vi "Read Instant Analog.vi"(10 "Channel":T1, 11 "ADALM2000 Handler":u64 caption="Instrument Handle Out") -> (2 "Read instant analog value":dbl(slide) max=255.0 scale=-25.0..25.0, 3 "ADALM2000 Handler 2":u64 caption="Instrument Handle Out")   [LabVIEW 2022 SP3]
uses:
  Controls/AnalogChannel.ctl
  libm2k_lv.dll
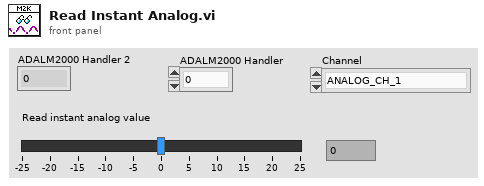
[diagram p1: front panel]
types:
  T1 = typedef "AnalogChannel.ctl" = enum16{"ANALOG_CH_1", "ANALOG_CH_2"}
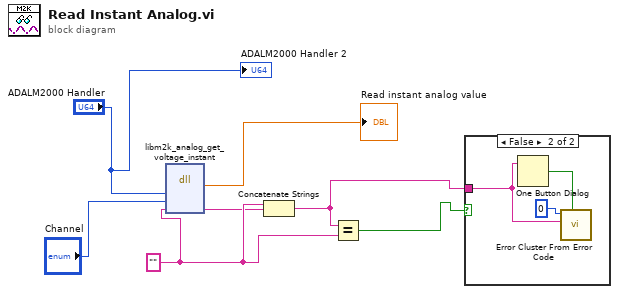
[diagram p0: block diagram]
diagram:
  w4 = ""
  n1 = dll-call lib="libm2k_lv.*" fn="libm2k_analog_get_voltage_instant"("instance"="ADALM2000 Handler", "chnIdx"="Channel", "err"=w4) -> ("return type"=→"Read instant analog value":dbl, "err"=w3:string)  [unwired: 5 in, 2 out]
  n2 = Concatenate Strings(w4, w3) -> (w6:string)
  n3 = Equal?(x=w6, y=w4) -> (x = y?=w7:bool)
  n4 = case shown="False" w7 {
    tunnel: w6 -> [_ w8]
    frame True {
    }
    frame False {
      n5 = One Button Dialog(message=w8) -> (true=w10:bool)  [unwired: 1 in]
      n6 = call <vilib>:"Error Cluster From Error Code.vi"("show call chain? (False)"=w10, "error message (\"\")"=w8, "error code (0)"=0) -> ()  [unwired: 6 in, 1 out]
    }
  }
  "ADALM2000 Handler 2" <- "ADALM2000 Handler"
